vi "Zaber Expert - Enter a List of Commands.vi"() -> ()   [LabVIEW 2020]
doc: "This example is more general purpose than the previous ones. It lets you enter a list of commands and then executes them, waiting for responses before sending the next command. If you send any commands to device 0 (All devices) or any group aliases, be sure to tell each command how many responses to wait for. This example is similar to the script editor in the Zaber Console.\nLabview features demonstrated here include autoindexed input from the Requests array, and a case structure around the Request (doesn't send after the quit button is clicked)."
uses:
  Public/Utility/Request.ctl
  Public/Utility/Response.ctl
  ZaberTSeries.lvlib
panel:
  out "Responses":T1[](array[typedef]) {"Command" items=["Constant Speed Tracking"=8, "Echo"=55, "Error"=255, "Home"=1, "Limit Active"=9, "Manual Move Tracking"=10, "Move Absolute"=20, "Move at Constant Speed"=22, "Move Relative"=21, "Renumber"=2, "Restore Settings"=36, "Stop"=23]}
  in  "Requests":T2[](array[typedef]) {"Command" items=["Echo"=55, "Home"=1, "Move Absolute"=20, "Move Relative"=21, "Move at Constant Speed"=22, "Renumber"=2, "Restore Settings"=36, "Stop"=23]}
  in  "Quit":bool
  in  "Go":bool
  in  "VISA resource name":refnum<visa-resource-name>
  # "Click the run arrow, select a COM port, enter a list of commands, and click Go. Each will\nexecute, waiting for responses before sending the next command. If you send commands to\ndevice 0 or aliases, specify how many responses to wait for.\nThis is similar to the script editor in the Zaber Console."
  # "Device, Command, Data, Response Count"
  # "Device, Command, Data"
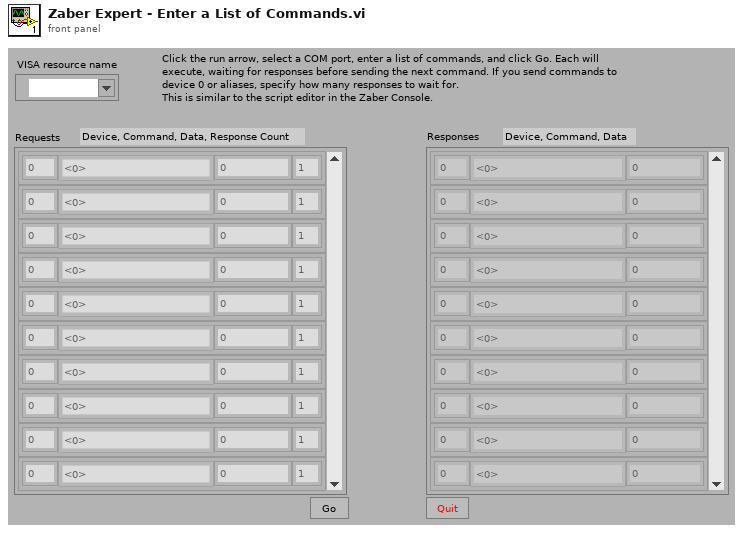
[diagram p1: front panel]
types:
  T1 = typedef "ZaberTSeries.lvlib/Response.ctl" = cluster{"Device Number":u8, "Command":u8, "Data":i32}
  T2 = typedef "ZaberTSeries.lvlib/Request.ctl" = cluster{"Device Number":u8, "Command":u8, "Data":i32, "Response Count":i32}
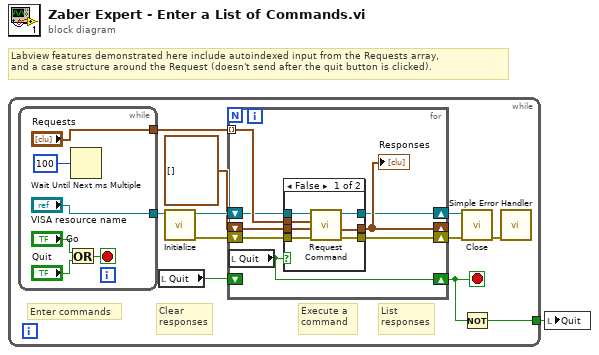
[diagram p0: block diagram]
diagram:
  # "Labview features demonstrated here include autoindexed input from the Requests array,\nand a case structure around the Request (doesn't send after the quit button is clicked)."
  n1 = while {
    tunnel: [w4] -> w1
    stop <- w5 stop-if-true
    # "List\nresponses"
    # "Execute a\ncommand"
    # "Clear\nresponses"
    # "Enter commands"
    n2 = while {
      tunnel: ["VISA resource name"] -> w12
      tunnel: ["Requests"] -> w10
      stop <- w34 stop-if-true
      n3 = Or(x="Go", y="Quit") -> (x .or. y?=w34:bool)
      n4 = Wait Until Next ms Multiple(millisecond multiple=u32 100) -> ()  [unwired: 1 out]
    }
    n5 = local read "Quit"() -> (w2:bool)
    n6 = call "Initialize.vi"("VISA resource name"=w12) -> ("error out"=w11:errorcluster, "VISA resource name out"=w6:refnum<visa-resource-name>)  [unwired: 8 in, 1 out]
    n7 = for {
      shift-right: [w20] -> _
      shift-left: T1[] [] ("Responses in") -> [w14]
      tunnel: w10 -> [w19] mode=indexing
      shift-right: [w18] -> w8
      shift-left: w11 -> [w16]
      shift-right: [w13] -> w5
      shift-left: w2 -> [_]
      shift-right: [w15] -> w7
      shift-left: w6 -> [w17]
      n8 = local read "Quit"() -> (w13:bool)
      n9 = case shown="False" w13 {
        tunnel: [w27 w29] -> w20
        tunnel: w19 -> [w26 _]
        tunnel: [w25 w28] -> w18
        tunnel: w17 -> [w24 w30]
        tunnel: w16 -> [w23 w28]
        tunnel: [w22 w30] -> w15
        tunnel: w14 -> [w21 w29]
        frame False {
          n10 = call "Request Command.vi"("error in (no error)"=w23, "Responses in"=w21, "Request"=w26, "VISA resource name"=w24) -> ("error out"=w25:errorcluster, "Responses out"=w27:T1[], "VISA resource name out"=w22:refnum<visa-resource-name>)  [unwired: 4 in, 1 out]
        }
        frame True {
        }
      }
      "Responses" <- w20
    }
    n11 = call "Close.vi"("error in (no error)"=w8, "VISA resource name"=w7) -> ("error out"=w9:errorcluster)  [unwired: 8 in, 1 out]
    n12 = Not(x=w5) -> (.not. x?=w4:bool)
    n13 = call <vilib>:"Simple Error Handler.vi"("error in (no error)"=w9) -> ()  [unwired: 4 in, 5 out]
  }
  n14 = local write "Quit"(w1) -> ()
